vi "MccHat_extract_data_02.vi"(8 "readings":cluster{i32, i32, dbl}[](array[cluster]), 11 "time":timestamp) -> (0 "temperature_array":dbl[](array[numeric]), 3 "waveform_array":waveform(dbl)[](array[waveform])=[{"t0"=timestamp(0 s since 1904-01-01), "dt"=1.0, "Y"=[]}, {"t0"=timestamp(3732035173.078092 s since 1904-01-01), "dt"=1.0, "Y"=[302.8589782714844], "attributes"=variant("NI_ChannelName"=variant(string "T1"))}])   [LabVIEW 2019]
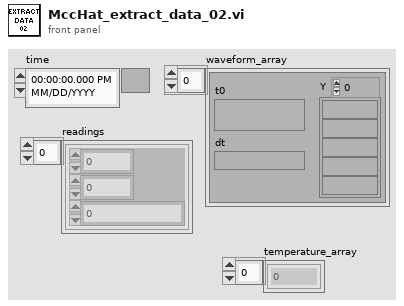
[diagram p1: front panel]
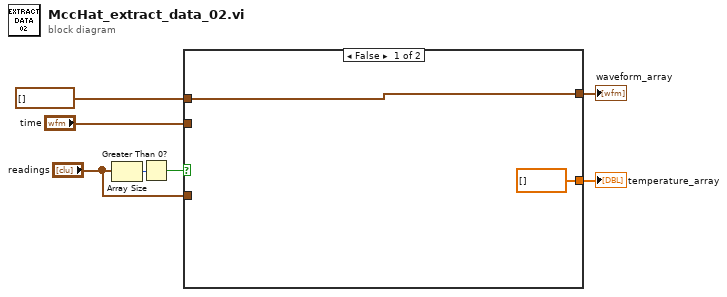
[diagram p0: block diagram]
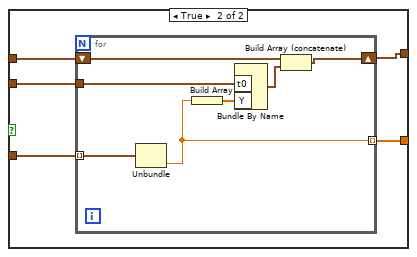
[diagram p2: hidden frame]
diagram:
  n1 = Array Size(array="readings") -> (size(s)=w3:i32)
  n2 = Greater Than 0?(x=w3) -> (x > 0?=w7:bool)
  n3 = case shown="False" w7 {
    tunnel: waveform(dbl)[] [] -> [w9 w14]
    tunnel: "time" -> [_ w13]
    tunnel: [w9 w12] -> w4
    tunnel: [dbl[] [] w10] -> w1
    tunnel: "readings" -> [_ w11]
    frame False {
    }
    frame True {
      n4 = for {
        tunnel: w13 -> [w20]
        tunnel: w11 -> [w15] mode=indexing
        tunnel: [w16] -> w10 mode=indexing
        shift-right: [w19] -> w12
        shift-left: w14 -> [w21]
        n5 = Unbundle(w15) -> (w16:dbl)  [unwired: 2 out]
        n6 = Build Array(w16) -> (w18:dbl[])
        n7 = Bundle By Name("t0"=w20, "Y"=w18) -> (w17:waveform(dbl))  [unwired: 1 in]
        n8 = Build Array (concatenate)(w21, w17) -> (w19:waveform(dbl)[])
      }
    }
  }
  "waveform_array" <- w4
  "temperature_array" <- w1
